vi "Vector_Plotting.vi"(1 "Template Filename":path, 2 "Data":string[][](array[string]), 3 "Channel Names":string[](array[string])) -> ()   [LabVIEW 2011]
uses:
  Globals/Constants_global.vi
  Controls/Group_Binning.ctl
  Data_File_Type.ctl
panel:
  in  "V":u16(ring) items=["Mode", "Turbine", "Azimuth", "X (mm)", "Y (mm)", "Z (mm)", "X refTurbine (m)", "Y refTurbine (m)", "Z refHub (m)", "Location", "Location Offset", "Uhf/Uref", "Turbulence hf (%)", "Vmag5hp/Uref (%)", "U5hp/Uref (%)", "V5hp/Uref (%)", "W5hp/Uref (%)", "Vmag 5hp (m/s)", "U 5hp (m/s)", "V 5hp (m/s)", "W 5hp (m/s)", "Lengthscale Estimate (m)", "Uref", "Uhw", "Variance HW", "HW (Uhw) Timescale Estimate Integrated to 25%", "HW (Uhw) Standard Error in Mean", "Notes", "ReturnType Plug in", "Date", "Start", "Time", "Seconds since 1st Jan", "Roughness Height", "Trip Height", "Comments", "Messages", "Current Data Filename", "Raw Data Filename", "Run Reject Reason", "Turbine X", "Turbine Y"]
  in  "U":u16(ring) items=["Mode", "Turbine", "Azimuth", "X (mm)", "Y (mm)", "Z (mm)", "X refTurbine (m)", "Y refTurbine (m)", "Z refHub (m)", "Location", "Location Offset", "Uhf/Uref", "Turbulence hf (%)", "Vmag5hp/Uref (%)", "U5hp/Uref (%)", "V5hp/Uref (%)", "W5hp/Uref (%)", "Vmag 5hp (m/s)", "U 5hp (m/s)", "V 5hp (m/s)", "W 5hp (m/s)", "Lengthscale Estimate (m)", "Uref", "Uhw", "Variance HW", "HW (Uhw) Timescale Estimate Integrated to 25%", "HW (Uhw) Standard Error in Mean", "Notes", "ReturnType Plug in", "Date", "Start", "Time", "Seconds since 1st Jan", "Roughness Height", "Trip Height", "Comments", "Messages", "Current Data Filename", "Raw Data Filename", "Run Reject Reason", "Turbine X", "Turbine Y"]
  in  "Y Axis":u16(ring) items=["Mode", "Turbine", "Azimuth", "X (mm)", "Y (mm)", "Z (mm)", "X refTurbine (m)", "Y refTurbine (m)", "Z refHub (m)", "Location", "Location Offset", "Uhf/Uref", "Turbulence hf (%)", "Vmag5hp/Uref (%)", "U5hp/Uref (%)", "V5hp/Uref (%)", "W5hp/Uref (%)", "Vmag 5hp (m/s)", "U 5hp (m/s)", "V 5hp (m/s)", "W 5hp (m/s)", "Lengthscale Estimate (m)", "Uref", "Uhw", "Variance HW", "HW (Uhw) Timescale Estimate Integrated to 25%", "HW (Uhw) Standard Error in Mean", "Notes", "ReturnType Plug in", "Date", "Start", "Time", "Seconds since 1st Jan", "Roughness Height", "Trip Height", "Comments", "Messages", "Current Data Filename", "Raw Data Filename", "Run Reject Reason", "Turbine X", "Turbine Y"]
  in  "X Axis":u16(ring) items=["Mode", "Turbine", "Azimuth", "X (mm)", "Y (mm)", "Z (mm)", "X refTurbine (m)", "Y refTurbine (m)", "Z refHub (m)", "Location", "Location Offset", "Uhf/Uref", "Turbulence hf (%)", "Vmag5hp/Uref (%)", "U5hp/Uref (%)", "V5hp/Uref (%)", "W5hp/Uref (%)", "Vmag 5hp (m/s)", "U 5hp (m/s)", "V 5hp (m/s)", "W 5hp (m/s)", "Lengthscale Estimate (m)", "Uref", "Uhw", "Variance HW", "HW (Uhw) Timescale Estimate Integrated to 25%", "HW (Uhw) Standard Error in Mean", "Notes", "ReturnType Plug in", "Date", "Start", "Time", "Seconds since 1st Jan", "Roughness Height", "Trip Height", "Comments", "Messages", "Current Data Filename", "Raw Data Filename", "Run Reject Reason", "Turbine X", "Turbine Y"]
  in  "OK Button":bool
  in  "Row Selector":i32(listbox)=1
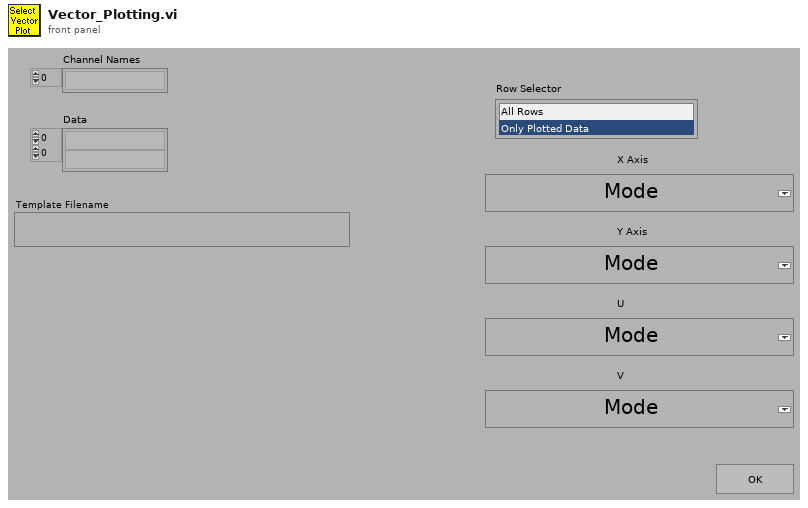
[diagram p1: front panel]
types:
  T1 = typedef "Data_File_Type.ctl" = enum16{"Read All File Types", "Results Files Only", "Raw Data Files Only", "Calibration Files Only", "Gas Desk Files Only", "Old Results Files Only", "Tabulated Data Files Only"}
  T2 = enum16{"Show only data summary", "Show data summary", "No data summary"}
  T3 = typedef "Group_Binning.ctl" = cluster{"Index":i32, "Tolerance":dbl, "Precision":string}
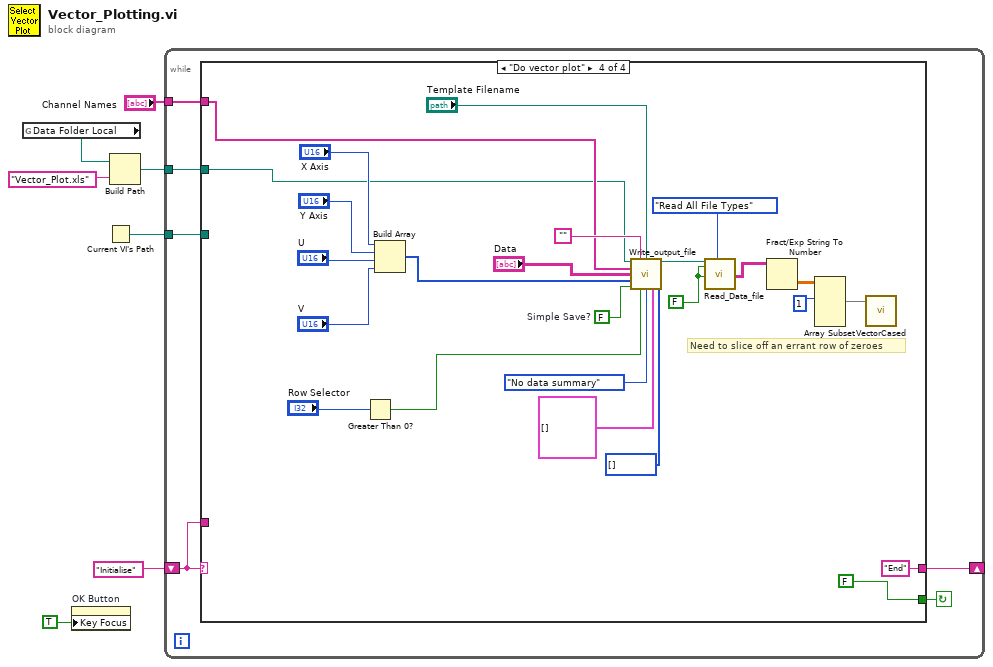
[diagram p0: block diagram]
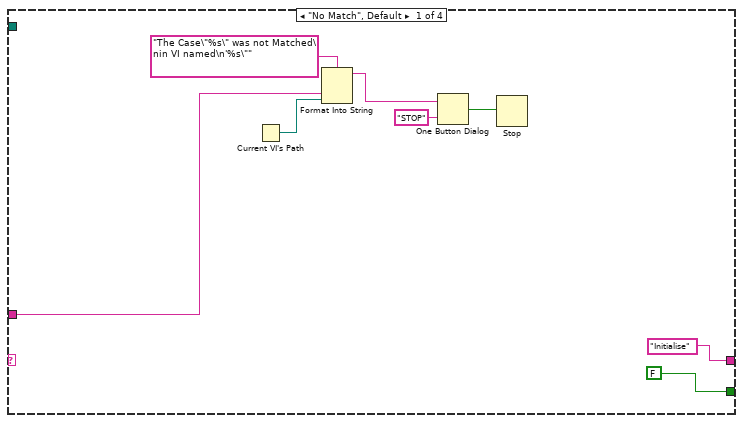
[diagram p2: hidden frame]
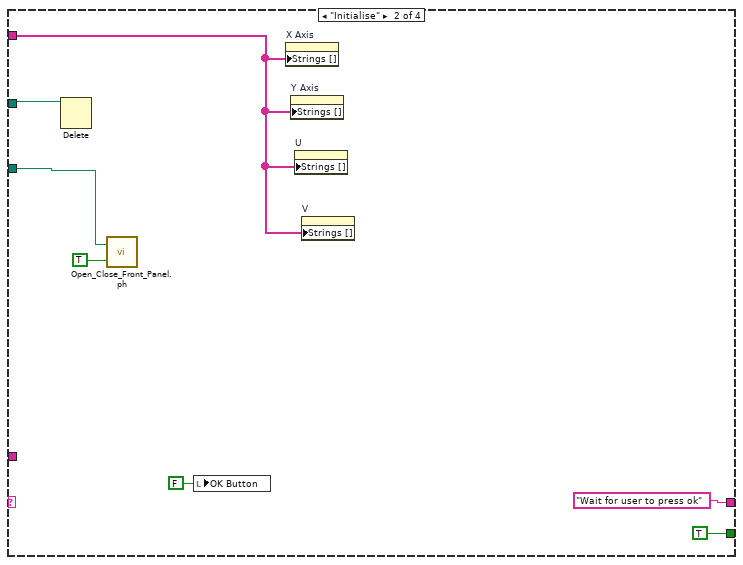
[diagram p3: hidden frame]
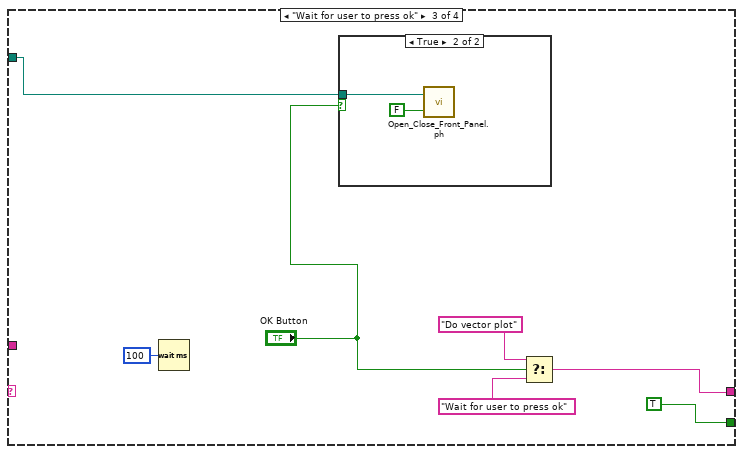
[diagram p4: hidden frame]
diagram:
  n1 = global read "Constants_global.vi" "Data Folder Local"() -> (w3:path)
  n2 = property on="OK Button" class="Bool (strict)"("Key Focus"=TRUE) -> ()  [unwired: 2 in, 2 out]
  n3 = Current VI's Path() -> (path=w6:path)
  n4 = Build Path(base path=w3, name or relative path="Vector_Plot.xls") -> (appended path=w1:path)
  n5 = while {
    shift-left: "Initialise" -> [w11]
    shift-right: [w12] -> _
    tunnel: w6 -> [w10]
    tunnel: "Channel Names" -> [w9]
    tunnel: w1 -> [w8]
    stop <- w13 continue-if-true
    n6 = case shown="\"Do vector plot\"" w11 {
      tunnel: [FALSE TRUE TRUE FALSE] -> w13
      tunnel: ["Initialise" "Wait for user to press ok" w34 "End" ("t")] -> w12
      tunnel: w11 -> [w16 _ _ _]
      tunnel: w10 -> [_ w26 w29 _]
      tunnel: w9 -> [_ w24 _ w43]
      tunnel: w8 -> [_ w22 _ w42]
      frame "No Match", Default {
        n7 = Current VI's Path() -> (path=w15:path)
        n8 = Format Into String(format string="The Case\"%s\" was not Matched\nin VI named\n'%s\"" ("Format String"), w16, w15) -> (resulting string=w19:string)  [unwired: 2 in, 1 out]
        n9 = One Button Dialog(message=w19, button name ("OK")="STOP") -> (true=w17:bool)
        n10 = Stop(stop? (T)=w17) -> ()
      }
      frame "Initialise" {
        n11 = Delete(path (use dialog)=w22) -> ()  [unwired: 1 in, 6 out]
        n12 = call "Open_Close_Front_Panel.ph.vi"("Front Panel Window:Open"=TRUE, "VI path"=w26) -> ()  [unwired: 2 out]
        n13 = local write "OK Button"(FALSE ("OK Button")) -> ()
        n14 = property on="X Axis" class="Ring (strict)"("Strings []"=w24) -> ()  [unwired: 2 in, 2 out]
        n15 = property on="Y Axis" class="Ring (strict)"("Strings []"=w24) -> ()  [unwired: 2 in, 2 out]
        n16 = property on="U" class="Ring (strict)"("Strings []"=w24) -> ()  [unwired: 2 in, 2 out]
        n17 = property on="V" class="Ring (strict)"("Strings []"=w24) -> ()  [unwired: 2 in, 2 out]
      }
      frame "Wait for user to press ok" {
        n18 = Wait (ms)(milliseconds to wait=u32 100) -> ()  [unwired: 1 out]
        n19 = case shown="True" "OK Button" {
          tunnel: w29 -> [_ w36]
          frame False {
          }
          frame True {
            n20 = call "Open_Close_Front_Panel.ph.vi"("Front Panel Window:Open"=FALSE, "VI path"=w36) -> ()  [unwired: 2 out]
          }
        }
        n21 = Select(t="Do vector plot", s="OK Button", f="Wait for user to press ok") -> (s? t:f=w34:string)
      }
      frame "Do vector plot" {
        w46 = FALSE ("Read Channel Names only")
        w55 = FALSE  # Simple Save?
        # "Need to slice off an errant row of zeroes"
        n22 = Greater Than 0?(x="Row Selector") -> (x > 0?=w56:bool)
        n23 = Build Array("X Axis", "Y Axis", "U", "V") -> (w50:u16[])
        n24 = call "Write_output_file.vi"("Output filename"=w42, "Header"="", "Template Filename"="Template Filename", "Channel Names"=w43, "Data"="Data", "Desired Columns"=w50, "Simple Save?"=w55, "Save Plotted rows only?"=w56, "Summarise mode"=T2."No data summary", "Grouping info"=T3[] [], "Channels to Tabulate in header"=i32[] []) -> ("Output filename Out"=w47:path)  [unwired: 1 in, 3 out]
        n25 = call "Read_Data_file.vi"("Results file"=w47, "Read Channel Names only"=w46, "Add Extra Channels?"=w46, "Desired File Types"=Data_File_Type."Read All File Types") -> ("Channel Values Out"=w44:string[][])  [unwired: 1 in, 14 out]
        n26 = Fract/Exp String To Number(string=w44) -> (number=w40:dbl[][])  [unwired: 4 out]
        n27 = Array Subset(array=w40, index (row)=1 ("index")) -> (w39:dbl[][])  [unwired: 3 in]
        n28 = call "VectorCased.vi"("XYUVArray"=w39) -> ()  [unwired: 11 out]
      }
    }
  }
